vi "_UpdateResTable.vi"(6 "CalResultIn":T1, 7 "Valid Peak?":bool, 8 "Resolution":dbl[][](array[numeric])=[[0.0, 0.0], [59.06, 8007.972231628852], [175.13, 24051.118700948115], [609.3, 84085.25564675158], [616.46, 85075.93195639057], [906.67, 125230.14589777726], [1254.9, 173425.601618889], [1487.09, 205562.74183429], [1500.0, 207349.59949474406]] format="%.2f", 9 "RefMass":dbl, 10 "FoundPW":dbl, 11 "Found":bool) -> (0 "ResolutionOut":dbl[][](array[numeric])=[[0.0, 0.0], [59.06, 8007.972231628852], [175.13, 24051.118700948115], [609.3, 84085.25564675158], [616.46, 85075.93195639057], [906.67, 125230.14589777726], [1254.9, 173425.601618889], [1487.09, 205562.74183429], [1500.0, 207349.59949474406]] format="%.2f", 1 "ResValid":bool, 2 "ResOK":bool, 3 "CalResultOut":T1, 4 "New DAC":dbl, 5 "ClosestIndex":i32)   [LabVIEW 2015]
uses:
  Type/_CalibrationResult.ctl
  Type/_Log Command.ctl
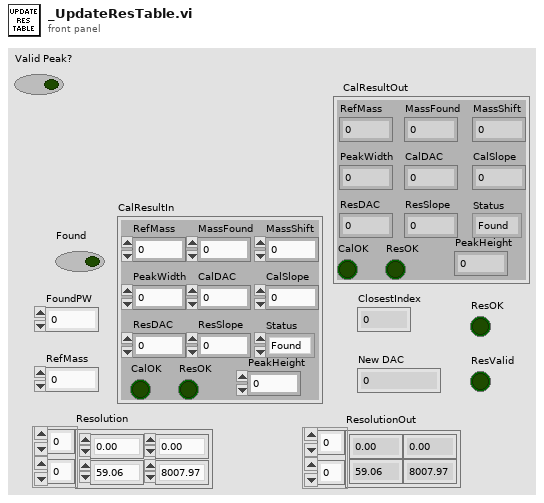
[diagram p1: front panel]
types:
  T1 = typedef "_CalibrationResult.ctl" = cluster{"RefMass":dbl, "MassFound":dbl, "MassShift":dbl, "PeakWidth":dbl, "CalDAC":dbl, "CalSlope":dbl, "ResDAC":dbl, "ResSlope":dbl, "Status":enum16{"Found", "Missing", "Not Used"}, "CalOK":bool, "ResOK":bool, "PeakHeight":dbl}
  T2 = typedef "_Log Command.ctl" = enum16{"No Command", "Open", "Read", "Write", "Close", "Check Size"}
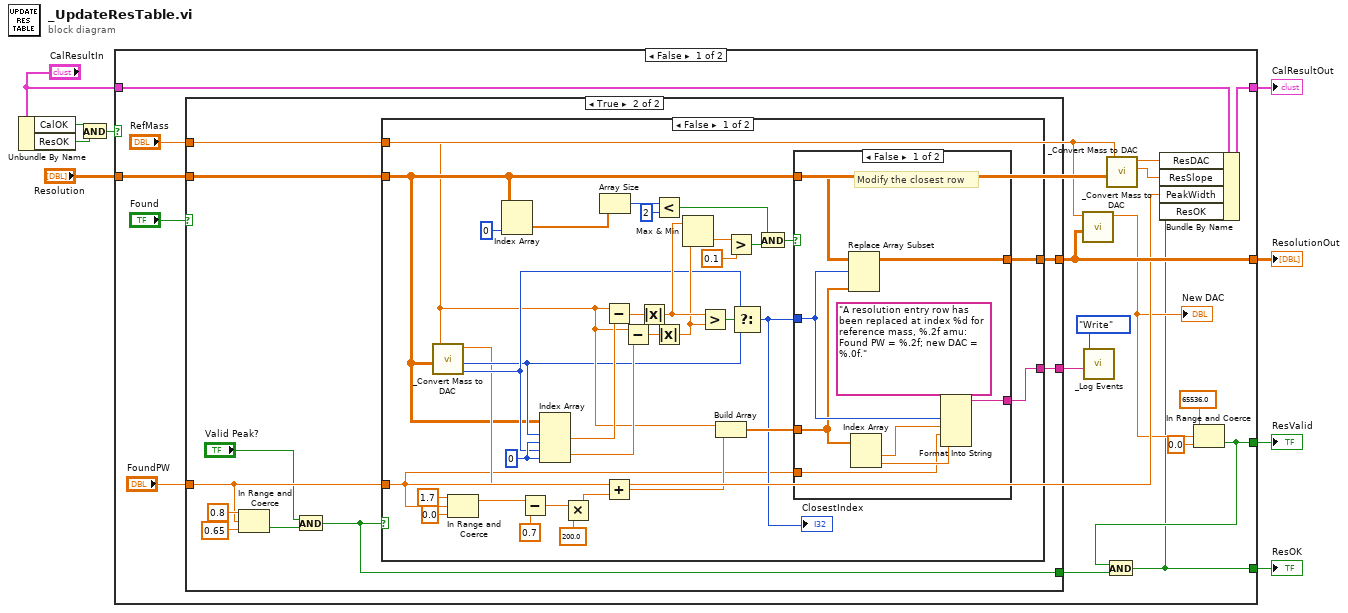
[diagram p0: block diagram]
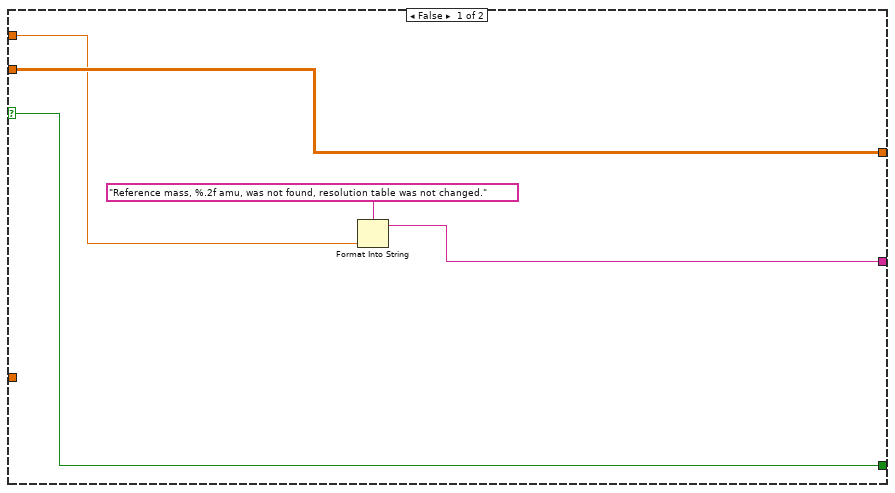
[diagram p2: hidden frame]
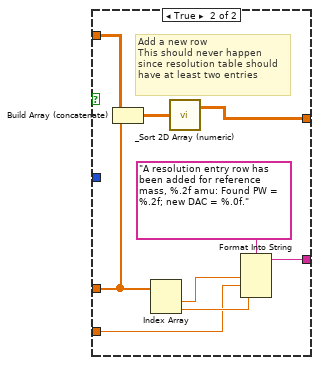
[diagram p3: hidden frame]
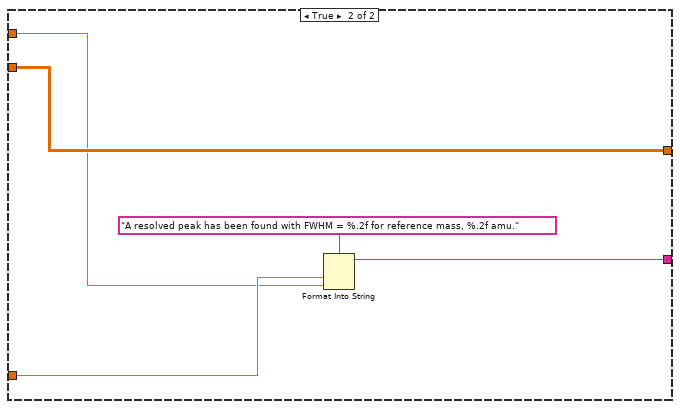
[diagram p4: hidden frame]
diagram:
  n1 = Unbundle By Name("CalResultIn") -> ("CalOK"=w2:bool, "ResOK"=w1:bool)
  n2 = And(x=w2, y=w1) -> (x .and. y?=w3:bool)
  n3 = case shown="False" w3 {
    selector: w3 -> [_ w100]
    tunnel: "Resolution" -> [w23 w101]
    tunnel: [w22 w101] -> w8
    tunnel: "CalResultIn" -> [w20 w102]
    tunnel: [w19 w102] -> w7
    tunnel: [w11 w100] -> w5
    tunnel: [w10 w100] -> w4
    frame False {
      n4 = case shown="True" "Found" {
        selector: "Found" -> [w27 _]
        tunnel: [w31 w41] -> w22
        tunnel: "RefMass" -> [w29 w40]
        tunnel: w23 -> [w31 w39]
        tunnel: [w28 w38] -> w24
        tunnel: "FoundPW" -> [_ w35]
        tunnel: [w27 w33] -> w12
        frame False {
          n5 = Format Into String(format string="Reference mass, %.2f amu, was not found, resolution table was not changed.", w29) -> (resulting string=w28:string)  [unwired: 2 in, 1 out]
        }
        frame True {
          n6 = In Range and Coerce(upper limit=0.8, x=w35, lower limit=0.65 ("upper limit")) -> (In Range?=w34:bool)  [unwired: 1 out]
          n7 = And(x="Valid Peak?", y=w34) -> (x .and. y?=w33:bool)
          n8 = case shown="False" w33 {
            tunnel: [w58 w99] -> w41
            tunnel: w40 -> [w57 w96]
            tunnel: w39 -> [w49 w99]
            tunnel: w35 -> [w44 w97]
            tunnel: [w56 w95] -> w38
            frame False {
              w76 = 0 ("disabled index (col)")
              n9 = call "_Convert Mass to DAC.vi"("Calibration Table"=w49, "Mass"=w57) -> ("LowerIndex"=w61:i32, "UpperIndex"=w55:i32, "DAC Value"=w52:dbl)  [unwired: 2 in, 1 out]
              n10 = In Range and Coerce(upper limit=1.7, x=w44, lower limit=0.0) -> (coerced(x)=w43:dbl)  [unwired: 1 out]
              n11 = Index Array(array=w49, index (col)=0 ("disabled index (col)")) -> (element=w48:dbl[])  [unwired: 1 in]
              n12 = Subtract(x=w43, y=0.7) -> (x-y=w53:dbl)
              n13 = Index Array(array=w49, index (row) #1=w55, index (col) #1=w76, index (row) #2=w61, index (col) #2=w76) -> (element #1=w75:dbl, element #2=w74:dbl)
              n14 = Multiply(x=w53, y=200.0) -> (x*y=w46:dbl)
              n15 = Array Size(array=w48) -> (size(s)=w66:i32)
              n16 = Subtract(x=w57, y=w75) -> (x-y=w73:dbl)
              n17 = Add(x=w52, y=w46) -> (x+y=w51:dbl)
              n18 = Subtract(x=w57, y=w74) -> (x-y=w72:dbl)
              n19 = Absolute Value(x=w73) -> (abs(x)=w70:dbl)
              n20 = Less?(x=w66, y=2) -> (x < y?=w63:bool)
              n21 = Absolute Value(x=w72) -> (abs(x)=w69:dbl)
              n22 = Max & Min(x=w70, y=w69) -> (min(x,y)=w68:dbl)  [unwired: 1 out]
              n23 = Greater?(x=w70, y=w69) -> (0:w71:bool)
              n24 = Build Array(w57, w51) -> (w60:dbl[])
              n25 = Greater?(x=w68, y=0.1) -> (0:w64:bool)
              n26 = Select(t=w61, s=w71, f=w55) -> (s? t:f=w59:i32)
              "ClosestIndex" <- w59
              n27 = And(x=w63, y=w64) -> (x .and. y?=w62:bool)
              n28 = case shown="False" w62 {
                tunnel: w49 -> [w85 w88]
                tunnel: w60 -> [w80 w87]
                tunnel: w59 -> [w82 _]
                tunnel: [w79 w86] -> w58
                tunnel: [w81 w92] -> w56
                tunnel: w44 -> [w77 w90]
                frame False {
                  # "Modify the closest row"
                  n29 = Replace Array Subset(array=w85, new element=w80, index (row)=w82) -> (w79:dbl[][])  [unwired: 1 in]
                  n30 = Index Array(array=w80) -> (element #1=w84:dbl, element #2=w78:dbl)  [unwired: 2 in]
                  n31 = Format Into String(format string="A resolution entry row has been replaced at index %d for reference mass, %.2f amu: Found PW = %.2f; new DAC = %.0f.", w82, w84, w77, w78) -> (resulting string=w81:string)  [unwired: 2 in, 1 out]
                }
                frame True {
                  # "Add a new row\nThis should never happen\nsince resolution table should\nhave at least two entries"
                  n32 = Build Array (concatenate)(w88, w87) -> (w89:dbl[][])
                  n33 = Index Array(array=w87) -> (element #1=w94:dbl, element #2=w91:dbl)  [unwired: 2 in]
                  n34 = call "_Sort 2D Array (numeric).vi"("Unsorted 2D Array"=w89) -> ("Sorted 2D Array"=w86:dbl[][])  [unwired: 4 in, 1 out]
                  n35 = Format Into String(format string="A resolution entry row has been added for reference mass, %.2f amu: Found PW = %.2f; new DAC = %.0f.", w94, w90, w91) -> (resulting string=w92:string)  [unwired: 2 in, 1 out]
                }
              }
            }
            frame True {
              n36 = Format Into String(format string="A resolved peak has been found with FWHM = %.2f for reference mass, %.2f amu.", w97, w96) -> (resulting string=w95:string)  [unwired: 2 in, 1 out]
            }
          }
        }
      }
      n37 = call "_Convert Mass to DAC.vi"("Calibration Table"=w22, "Mass"="RefMass") -> ("DAC Value"=w13:dbl)  [unwired: 2 in, 3 out]
      "New DAC" <- w13
      n38 = call "_Log Events.vi"("Event"=w24, "Log Command"=_Log_Command."Write") -> ()  [unwired: 6 in, 2 out]
      n39 = call "_Convert Mass to DAC.vi"("Calibration Table"=w23, "Mass"="RefMass") -> ("Slope"=w17:dbl, "DAC Value"=w18:dbl)  [unwired: 2 in, 2 out]
      n40 = In Range and Coerce(upper limit=65536.0, x=w13, lower limit=0.0) -> (In Range?=w11:bool)  [unwired: 1 out]
      n41 = And(x=w11, y=w12) -> (x .and. y?=w10:bool)
      n42 = Bundle By Name(cluster=w20, "ResDAC"=w18, "ResSlope"=w17, "PeakWidth"="FoundPW", "ResOK"=w10) -> (w19:T1)
    }
    frame True {
      # "The given reference peak has met the resolution criteria from the previous iteration.\nNo further adjustment required."
    }
  }
  "ResolutionOut" <- w8
  "CalResultOut" <- w7
  "ResOK" <- w4
  "ResValid" <- w5
